vi "Page_Advanced_WriteAll.vi"(6 "ctl references":T1, 8 "error in (no error)":errorcluster, 11 "AB_Build in":refnum<class "AB_Build.lvclass">) -> (0 "error out":errorcluster, 3 "AB_Build out":refnum<class "AB_Build.lvclass">)   [LabVIEW 2020, in "AB_Build.lvclass"]
uses:
  <vilib>/AppBuilder/AB_Classes/Build/AB_Build.lvclass
  <resource>/Framework/Providers/Builds/AppBuilder/AB_UI_Page_Advanced_References.ctl
  <vilib>/AppBuilder/AB_Classes/Build/AB_Build.lvclass/AB_Build.ctl
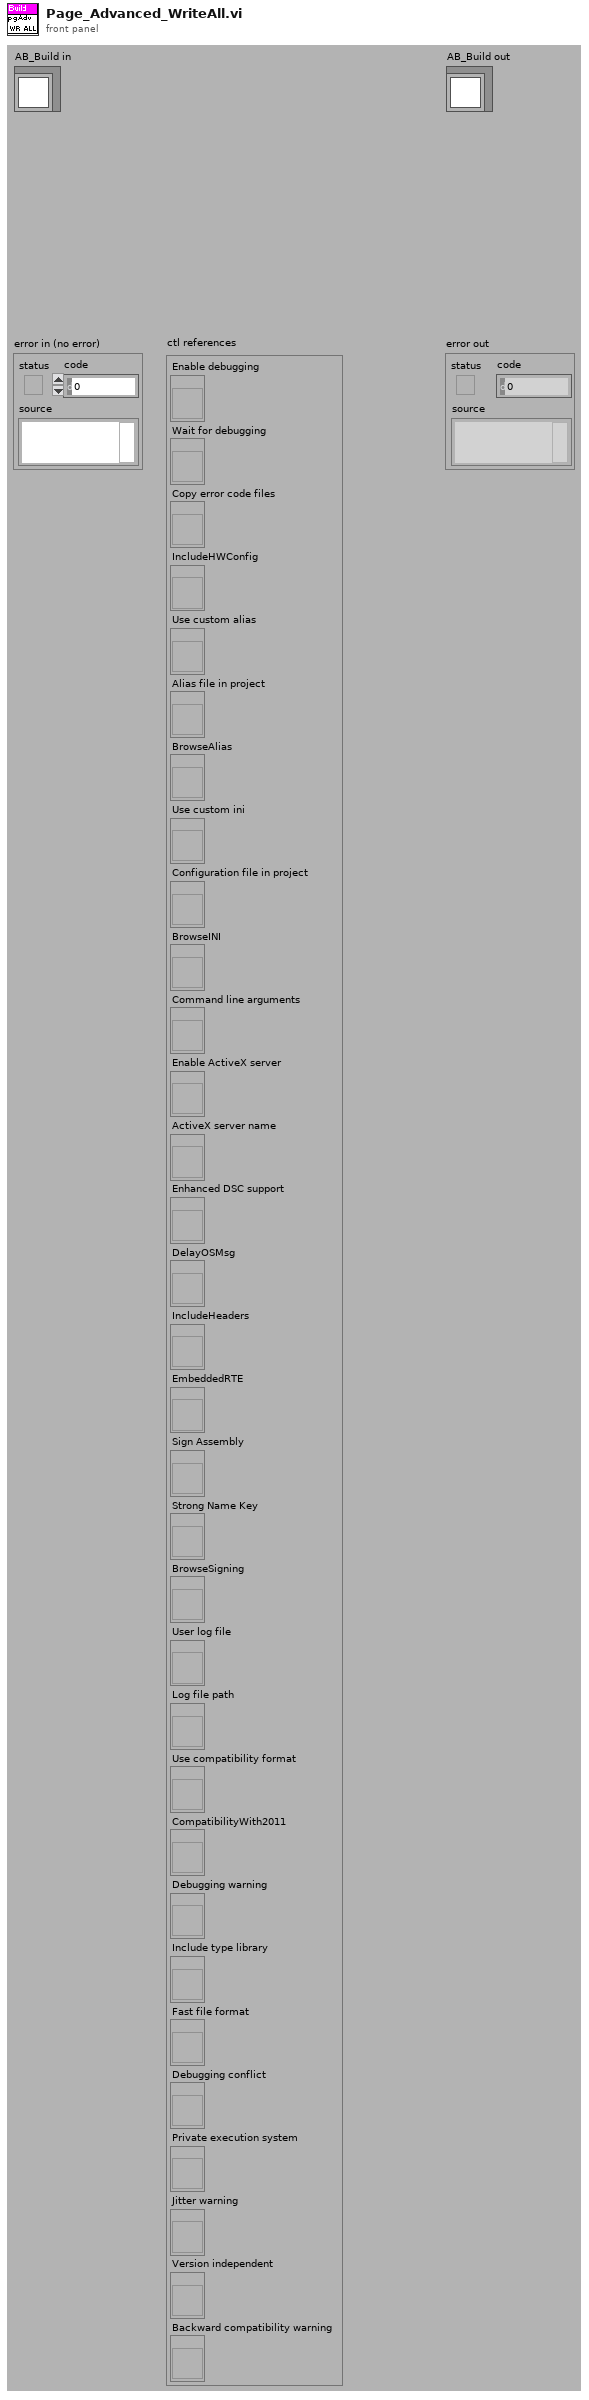
[diagram p1: front panel]
types:
  T1 = typedef "AB_UI_Page_Advanced_References.ctl" = cluster{"Enable debugging":refnum<vi>, "Wait for debugging":refnum<vi>, "Copy error code files":refnum<vi>, "IncludeHWConfig":refnum<vi>, "Use custom alias":refnum<vi>, "Alias file in project":refnum<vi>, "BrowseAlias":refnum<vi>, "Use custom ini":refnum<vi>, "Configuration file in project":refnum<vi>, "BrowseINI":refnum<vi>, "Command line arguments":refnum<vi>, "Enable ActiveX server":refnum<vi>, "ActiveX server name":refnum<vi>, "Enhanced DSC support":refnum<vi>, "DelayOSMsg":refnum<vi>, "IncludeHeaders":refnum<vi>, "EmbeddedRTE":refnum<vi>, "Sign Assembly":refnum<vi>, "Strong Name Key":refnum<vi>, "BrowseSigning":refnum<vi>, "User log file":refnum<vi>, "Log file path":refnum<vi>, "Use compatibility format":refnum<vi>, "CompatibilityWith2011":refnum<vi>, "Debugging warning":refnum<vi>, "Include type library":refnum<vi>, "Fast file format":refnum<vi>, "Debugging conflict":refnum<vi>, "Private execution system":refnum<vi>, "Jitter warning":refnum<vi>, "Version independent":refnum<vi>, "Backward compatibility warning":refnum<vi>}
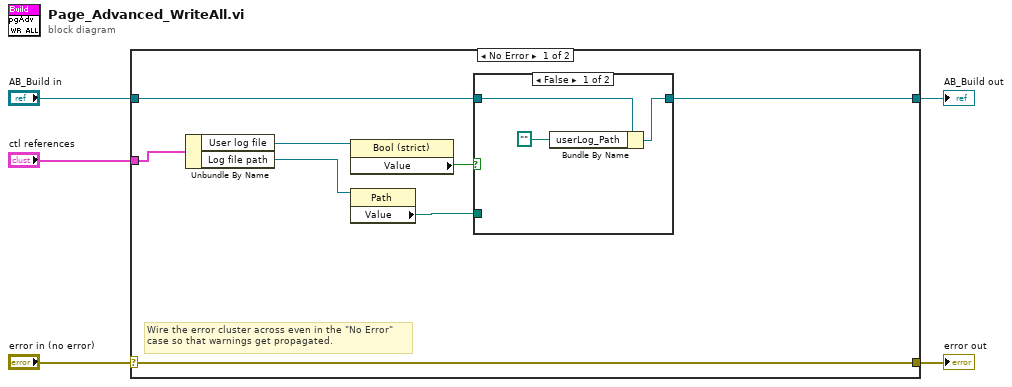
[diagram p0: block diagram]
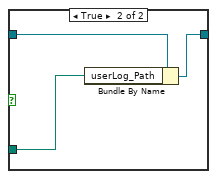
[diagram p2: hidden frame]
diagram:
  n1 = case shown="No Error" "error in (no error)" {
    selector: "error in (no error)" -> [w13 w21]
    tunnel: [w13 w21] -> w4
    tunnel: [w6 w20] -> w2
    tunnel: "AB_Build in" -> [w10 w20]
    tunnel: "ctl references" -> [w12 _]
    frame No Error {
      # "Wire the error cluster across even in the \"No Error\"\ncase so that warnings get propagated."
      n2 = Unbundle By Name(w12) -> ("User log file"=w11:refnum<vi>, "Log file path"=w8:refnum<vi>)
      n3 = property class="Bool (strict)"(reference=w11) -> ("Value"=w9:bool)  [unwired: 1 in, 2 out]
      n4 = property class="Path"(reference=w8) -> ("Value"=w7:path)  [unwired: 1 in, 2 out]
      n5 = case shown="False" w9 {
        tunnel: w10 -> [w16 w19]
        tunnel: w7 -> [_ w18]
        tunnel: [w15 w17] -> w6
        frame False {
          n6 = Bundle By Name(cluster=w16, "userLog_Path"=path "") -> (w15:refnum<class "AB_Build.lvclass">)
        }
        frame True {
          n7 = Bundle By Name(cluster=w19, "userLog_Path"=w18) -> (w17:refnum<class "AB_Build.lvclass">)
        }
      }
    }
    frame Error {
    }
  }
  "error out" <- w4
  "AB_Build out" <- w2
